vi "Get COB-ID.vi"(11 "CANopen Message in":refnum<class "CANopen Message.lvclass">) -> (2 "COB-ID":u32 format="%.0x", 3 "CANopen Message out":refnum<class "CANopen Message.lvclass">)   [LabVIEW 2024, in "CANopen Master.lvlib" / "CANopen Message.lvclass"]
uses:
  CANopen Message.lvclass
  CANopen Message.lvclass/CANopen Message.ctl
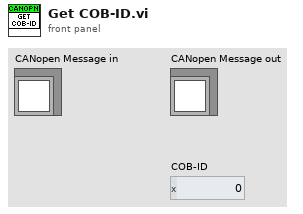
[diagram p1: front panel]
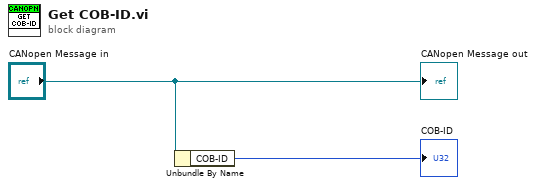
[diagram p0: block diagram]
diagram:
  n1 = Unbundle By Name("CANopen Message in") -> ("COB-ID"=→"COB-ID":u32)
  "CANopen Message out" <- "CANopen Message in"
